vi "SysDef.CreateWaveform.vi"(7 "GUID (Default Waveform)":string="83F792DC-AED3-09DF-CB38-512C04DA274D", 8 "error in (no error)":errorcluster, 9 "Waveform":T1, 10 "Name":string, 11 "nodeID":u64) -> (0 "error out":errorcluster, 1 "New NodeID":u64, 2 "newItem":bool, 3 "nodeID out":u64)   [LabVIEW 2015, in "Advanced System Definition.lvlib"]
uses:
  Advanced System Definition.lvlib
  <vilib>/NI Veristand/Custom Device API/Custom Device Waveform.ctl
  <vilib>/NI Veristand/Custom Device API/Custom Device Waveform DataType.ctl
  NationalInstruments.VeriStand.SystemDefinitionAPI
  <vilib>/NI Veristand/Custom Device API/Custom Device API.lvlib
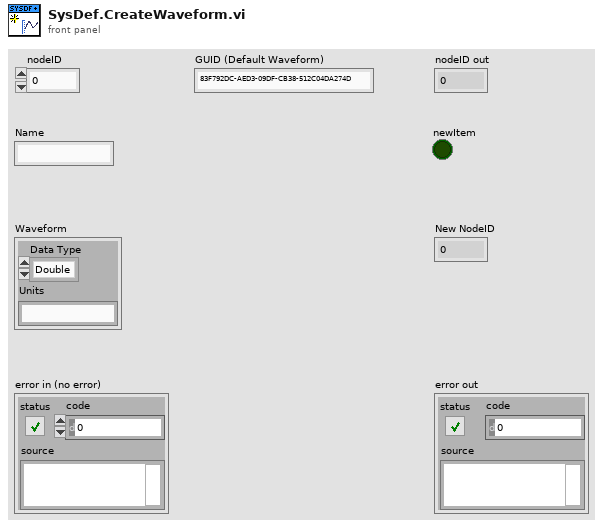
[diagram p1: front panel]
types:
  T1 = typedef "Custom Device API.lvlib/Custom Device Waveform.ctl" = cluster{"Data Type":T2, "Units":string}
  T2 = typedef "Custom Device API.lvlib/Custom Device Waveform DataType.ctl" = enum16{"Double", "Complex Double"}
  T3 = typedef "Custom Device API.lvlib/Custom Device Item Ref.ctl" = u64
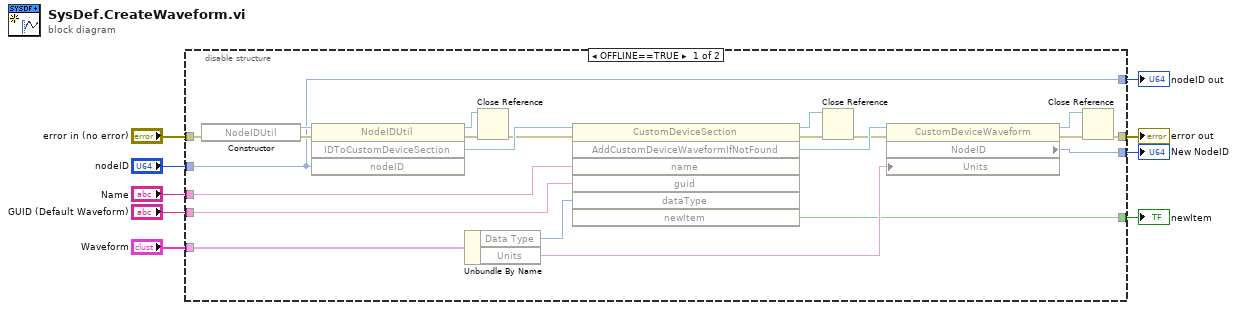
[diagram p0: block diagram]
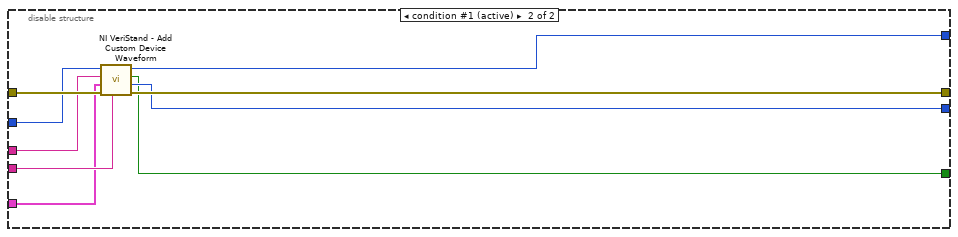
[diagram p2: hidden frame]
diagram:
  n1 = disable-structure shown="OFFLINE==TRUE" {
    disable-tunnel: "nodeID" -> [w10 w39]
    disable-tunnel: "error in (no error)" -> [w28 w40]
    disable-tunnel: [w27 w34] -> w8
    disable-tunnel: "Waveform" -> [w26 w36]
    disable-tunnel: "Name" -> [w25 w38]
    disable-tunnel: "GUID (Default Waveform)" -> [w24 w37]
    disable-tunnel: [w12 w35] -> w4
    disable-tunnel: [w11 w33] -> w3
    disable-tunnel: [w10 w32] -> w1
    frame condition #0 {
      n2 = constructor class="NodeIDUtil"(error in=w28) -> (reference out=w30:refnum<k24>, error out=w29:errorcluster)  [unwired: 2 in, 1 out]
      n3 = invoke class="NodeIDUtil" method="IDToCustomDeviceSection"(reference=w30, error in=w29, "nodeID"=w10) -> (reference out=w13:refnum<k24>, error out=w15:errorcluster, "IDToCustomDeviceSection"=w31:refnum<k24>)  [unwired: 1 in, 1 out]
      n4 = Unbundle By Name(w26) -> ("Data Type"=w19:T2, "Units"=w16:string)
      n5 = Close Reference(reference=w13, error in (no error)=w15) -> (error out=w14:errorcluster)
      n6 = invoke class="CustomDeviceSection" method="AddCustomDeviceWaveformIfNotFound"(reference=w31, error in=w14, "name"=w25, "guid"=w24, "dataType"=w19) -> (reference out=w22:refnum<k24>, error out=w23:errorcluster, "AddCustomDeviceWaveformIfNotFound"=w21:refnum<k24>, "newItem"=w11:bool)  [unwired: 2 in, 3 out]
      n7 = Close Reference(reference=w22, error in (no error)=w23) -> (error out=w20:errorcluster)
      n8 = property class="CustomDeviceWaveform"(reference=w21, error in=w20, "Units"=w16) -> (reference out=w18:refnum<k24>, error out=w17:errorcluster, "NodeID"=w27:u64)
      n9 = Close Reference(reference=w18, error in (no error)=w17) -> (error out=w12:errorcluster)
    }
    frame condition #1 (active) {
      n10 = call <vilib>:"NI VeriStand - Add Custom Device Waveform.vi"("GUID (Default Waveform)"=w37, "error in (no error)"=w40, "Waveform"=w36, "Waveform Name"=w38, "Parent Ref in"=w39) -> ("error out"=w35:errorcluster, "Waveform Ref"=w34:T3, "Newly Created?"=w33:bool, "Parent Ref out"=w32:T3)  [unwired: 3 in]
    }
  }
  "New NodeID" <- w8
  "nodeID out" <- w1
  "error out" <- w4
  "newItem" <- w3
